vi "Spectrograph_getEvent_errorCode.vi"(8 "error in (no error)":errorcluster, 11 "logevent_errorCode_Ctl":T1) -> (0 "error out":errorcluster, 2 "function return":i32, 3 "logevent_errorCode_Ctl out":T1)   [LabVIEW 2016, in "SALLV_Spectrograph.lvlib"]
doc: "int Spectrograph_shm_getEvent_errorCodeLV(Spectrograph_logevent_errorCodeLV *logevent_errorCode_Ctl );"
uses:
  SALLV_Spectrograph.lvlib
  DataTypes/logevent_errorCode.ctl
  SALLV_Spectrograph.so
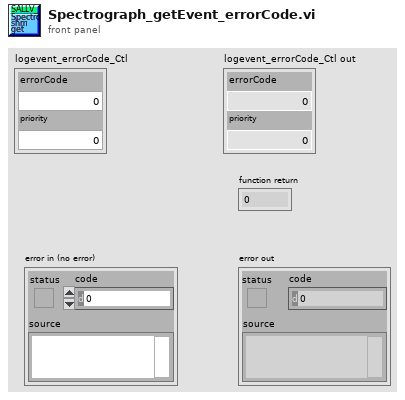
[diagram p1: front panel]
types:
  T1 = typedef "SALLV_Spectrograph.lvlib/logevent_errorCode.ctl" = cluster{"errorCode":i32, "priority":i32}
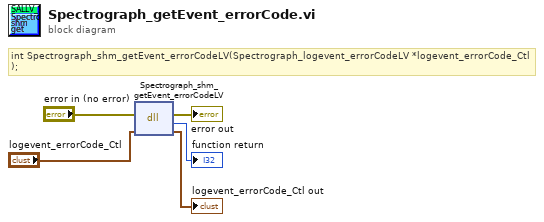
[diagram p0: block diagram]
diagram:
  # "int Spectrograph_shm_getEvent_errorCodeLV(Spectrograph_logevent_errorCodeLV *logevent_errorCode_Ctl );"
  n1 = dll-call lib="home/harini/TCS/SALLV_Spectrograph/SALLV_Spectrograph.*" fn="Spectrograph_shm_getEvent_errorCodeLV"(error in="error in (no error)", "logevent_errorCode_Ctl"="logevent_errorCode_Ctl") -> (error out=→"error out":errorcluster, →"function return":i32, "logevent_errorCode_Ctl"=→"logevent_errorCode_Ctl out":T1)  [unwired: 2 in, 1 out]
